vi "FGV Read PV Monitors.vi"(8 "Error In":errorcluster, 9 "CS++PVMonitor":refnum<class "CS++PVMonitor.lvclass">, 10 "PV Monitor":string) -> (0 "Error Out":errorcluster, 1 "CS++PVMonitor":refnum<class "CS++PVMonitor.lvclass">, 2 "Success":bool, 4 "PV Monitors":string[](array[string]), 6 "PVMonitors":refnum<class "CS++PVMonitor.lvclass">[](array[class]))   [LabVIEW 2015, in "CS++Base.lvlib"]
doc: "Read FGV maintaining a list of PV Monitor classes."
uses:
  CS++Base.lvlib
  Actors/CS++PVMonitor/CS++PVMonitor.lvclass
  FGV Action.ctl
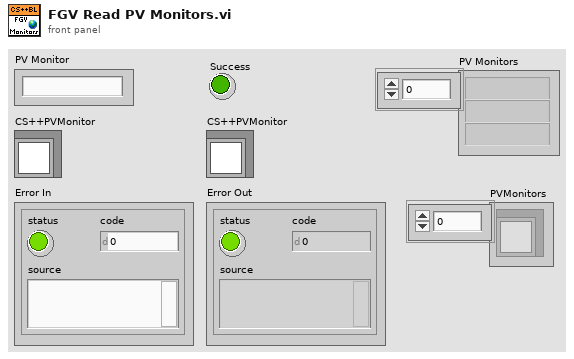
[diagram p1: front panel]
types:
  T1 = typedef "CS++Base.lvlib/FGV Action.ctl" = enum16{"add", "replace", "read", "remove", "reset", "get attributes"}
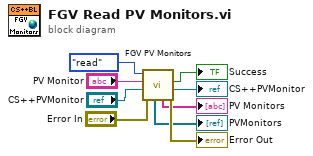
[diagram p0: block diagram]
diagram:
  n1 = call "FGV PV Monitors.vi"("Error In"="Error In", "CS++PVMonitor"="CS++PVMonitor", "PV Monitor"="PV Monitor", "Action (read)"=FGV_Action."read") -> ("Error Out"=→"Error Out":errorcluster, "CS++PVMonitor"=→"CS++PVMonitor":refnum<class "CS++PVMonitor.lvclass">, "Success"=→"Success":bool, "PV Monitors"=→"PV Monitors":string[], "PVMonitors"=→"PVMonitors":refnum<class "CS++PVMonitor.lvclass">[])  [unwired: 3 in]
